vi "string occurance.vi"() -> ()   [LabVIEW 2012]
panel:
  out "String 2":string
  out "Numeric":i16
  in  "search string":string
  in  "Array 2":string[](array[string])
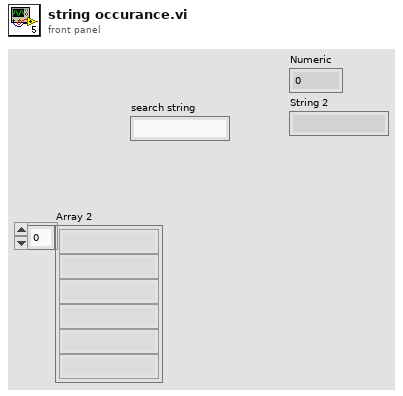
[diagram p1: front panel]
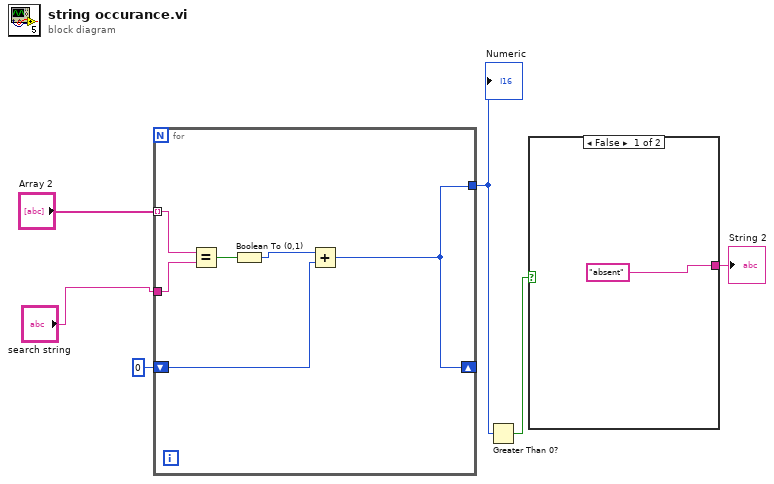
[diagram p0: block diagram]
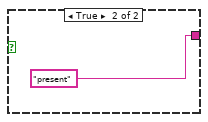
[diagram p2: hidden frame]
diagram:
  n1 = for {
    tunnel: "Array 2" -> [w12] mode=indexing
    tunnel: "search string" -> [w11]
    shift-right: [w7] -> _
    shift-left: i16 0 -> [w8]
    tunnel: [w7] -> w3
    n2 = Equal?(x=w12, y=w11) -> (x = y?=w10:bool)
    n3 = Boolean To (0,1)(Boolean=w10) -> (0, 1=w9:i16)
    n4 = Add(x=w9, y=w8) -> (x+y=w7:i16)
  }
  "Numeric" <- w3
  n5 = Greater Than 0?(x=w3) -> (x > 0?=w2:bool)
  n6 = case shown="False" w2 {
    tunnel: ["absent" "present"] -> w1
    frame False {
    }
    frame True {
    }
  }
  "String 2" <- w1
